vi "Initialize.vi"(8 "error in (no error)":errorcluster, 9 "Reset (True)":bool=TRUE, 10 "ID Query (True)":bool=TRUE, 11 "VISA resource name":refnum<visa-resource-name>) -> (0 "error out":errorcluster, 3 "VISA resource name out":refnum<visa-resource-name>)   [LabVIEW 2013, in "Template - Register.lvlib"]
doc: "Establishes communication with the instrument and optionally performs an instrument identification query and/or an instrument reset. It also places the instrument in a default state needed for other instrument driver operations. Therefore, call this VI before calling other instrument driver VIs for this instrument. Generally, you need to call the Initialize VI only once at the beginning of an application."
uses:
  <instrlib>/_Template - Register/Template - Register.lvlib
panel:
  # "(c) 2007 <Enter Company Name Here>.  ALL RIGHTS RESERVED."
  # "EDIT: Change control description to remove example text for buses not supported."
  # "EDIT: If your instrument does not support ID query or Reset, remove the ID Query or Reset control from the front panel and delete the case structure with the ID Query or Reset code from the block diagram."
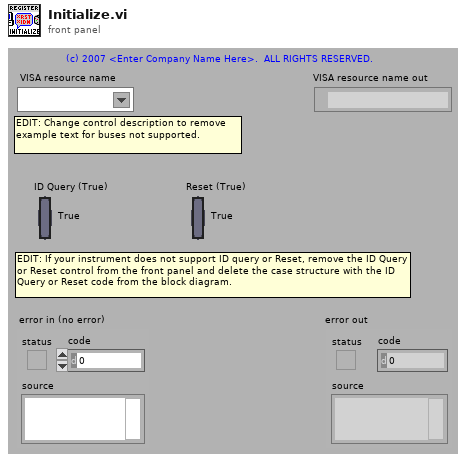
[diagram p1: front panel]
types:
  T1 = cluster{"Status":bool, "Code":i32, "Source (VI Name)":string}
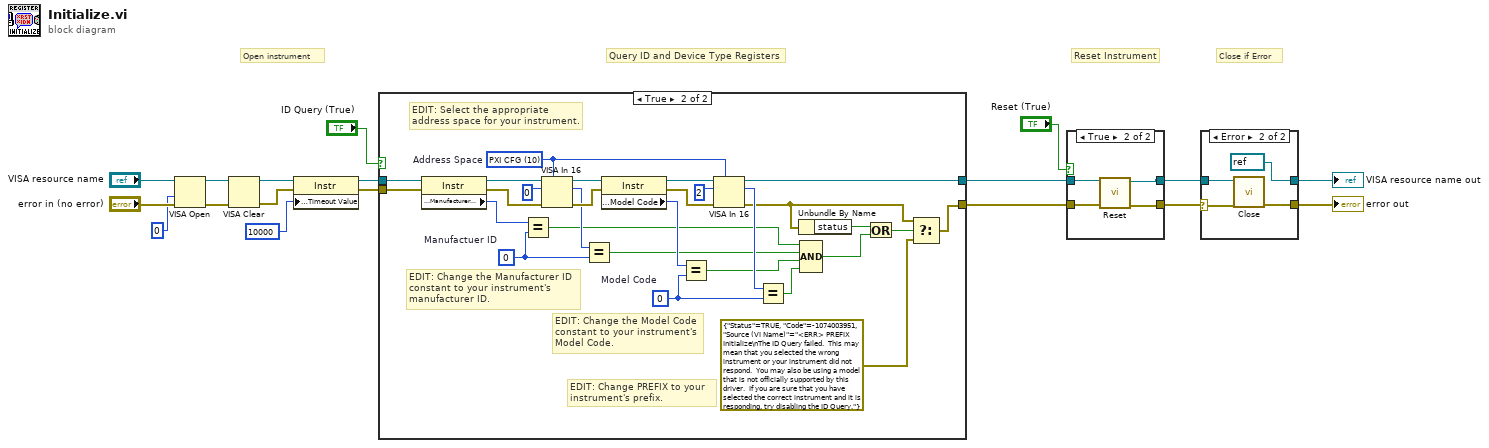
[diagram p0: block diagram]
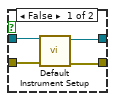
[diagram p3: hidden frame]
diagram:
  # "Close if Error"
  # "Query ID and Device Type Registers"
  # "Reset Instrument"
  # "Open instrument"
  n1 = VISA Open(access mode=u32 0, error in (no error)="error in (no error)", VISA resource name="VISA resource name") -> (VISA resource name=w4:refnum<visa-resource-name>, error out=w5:errorcluster)  [unwired: 2 in]
  n2 = VISA Clear(VISA resource name=w4, error in (no error)=w5) -> (VISA resource name out=w7:refnum<visa-resource-name>, error out=w6:errorcluster)
  n3 = property class="Instr"(reference=w7, error in=w6, "General Settings:Timeout Value"=u32 10000 ("Tmo Value")) -> (reference out=w8:refnum<visa-resource-name>, error out=w9:errorcluster)
  n4 = case shown="True" "ID Query (True)" {
    tunnel: [w20 w48] -> w18
    tunnel: w9 -> [w20 w45]
    tunnel: [w19 w34] -> w11
    tunnel: w8 -> [w19 w33]
    frame False {
    }
    frame True {
      w28 = u16 10 items=["A16"=1, "A24"=2, "A32"=3, "PXI CFG"=10, "PXI BAR0"=11, "PXI BAR1"=12, "PXI BAR2"=13, "PXI BAR3"=14, "PXI BAR4"=15, "PXI BAR5"=16]  # Address Space
      w40 = u16 0  # Manufactuer ID
      w32 = u16 0  # Model Code
      # "EDIT: Select the appropriate\naddress space for your instrument."
      # "EDIT: Change PREFIX to your\ninstrument's prefix."
      # "EDIT: Change the Model Code\nconstant to your instrument's\nModel Code."
      # "EDIT: Change the Manufacturer ID\nconstant to your instrument's\nmanufacturer ID."
      n5 = property class="Instr"(reference=w33, error in=w45) -> (reference out=w21:refnum<visa-resource-name>, error out=w44:errorcluster, "General Settings:Manufacturer Identification"=w47:u16)
      n6 = Equal?(x=w47, y=w40) -> (x = y?=w24:bool)
      n7 = VISA In 16(7:w28, 8:w44, 10:u32 0 ("offset (0)"), 11:w21) -> (0:w41:errorcluster, 2:w39:u16, 3:w42:refnum<visa-resource-name>)
      n8 = Equal?(x=w39, y=w40) -> (x = y?=w25:bool)
      n9 = property class="Instr"(reference=w42, error in=w41) -> (reference out=w38:refnum<visa-resource-name>, error out=w37:errorcluster, "General Settings:Model Code"=w46:u16)
      n10 = Equal?(x=w46, y=w32) -> (x = y?=w26:bool)
      n11 = VISA In 16(7:w28, 8:w37, 10:u32 2 ("offset (0)"), 11:w38) -> (0:w29:errorcluster, 2:w36:u16, 3:w34:refnum<visa-resource-name>)
      n12 = Equal?(x=w36, y=w32) -> (x = y?=w27:bool)
      n13 = Unbundle By Name(w29) -> ("status"=w30:bool)
      n14 = Compound Arithmetic op=AND(w24, w25, w26, w27) -> (w23:bool)
      n15 = Or(x=w30, y=w23) -> (x .or. y?=w31:bool)
      n16 = Select(t=w29, s=w31, f=T1 {"Status"=TRUE, "Code"=-1074003951, "Source (VI Name)"="<ERR> PREFIX Initialize\nThe ID Query failed.  This may mean that you selected the wrong instrument or your instrument did not respond.  You may also be using a model that is not officially supported by this driver.  If you are sure that you have selected the correct instrument and it is responding, try disabling the ID Query."}) -> (s? t:f=w48:T1)
    }
  }
  n17 = case shown="True" "Reset (True)" {
    tunnel: w18 -> [w51 w53]
    tunnel: [w49 w55] -> w2
    tunnel: [w50 w56] -> w3
    tunnel: w11 -> [w52 w54]
    frame False {
      n18 = call <instrlib>:"Default Instrument Setup.vi"("error in (no error)"=w51, "VISA resource name"=w52) -> ("error out"=w49:errorcluster, "VISA resource name out"=w50:refnum<visa-resource-name>)  [unwired: 8 in]
    }
    frame True {
      n19 = call <instrlib>:"Reset.vi"("error in (no error)"=w53, "VISA resource name"=w54) -> ("error out"=w55:errorcluster, "VISA resource name out"=w56:refnum<visa-resource-name>)  [unwired: 8 in]
    }
  }
  n20 = case shown="Error" w2 {
    selector: w2 -> [w57 w60]
    tunnel: [w57 w62] -> w12
    tunnel: w3 -> [w58 w61]
    tunnel: [w58 refnum<visa-resource-name> refnum ("VISA resource name out 2")] -> w13
    frame No Error {
    }
    frame Error {
      n21 = call <instrlib>:"Close.vi"("error in (no error)"=w60, "VISA resource name"=w61) -> ("error out"=w62:errorcluster)  [unwired: 9 in]
    }
  }
  "VISA resource name out" <- w13
  "error out" <- w12
